vi "Serial Port Clear v0.3.vi"(0 "Serial Port In":i32(ring) items=["Modem Port", "Printer Port", "Serial Card Port #1", "Serial Card Port #2", "Serial Card Port #3", "Serial Card Port #4"]) -> (1 "Serial Port Out":i32(ring) items=["Modem Port", "Printer Port", "Serial Card Port #1", "Serial Card Port #2", "Serial Card Port #3", "Serial Card Port #4"], 2 "string read":string)   [LabVIEW 2020]
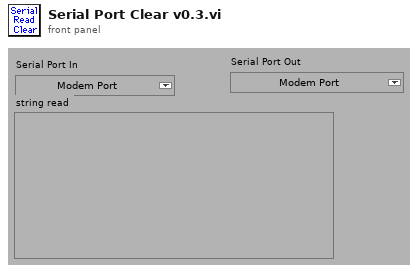
[diagram p1: front panel]
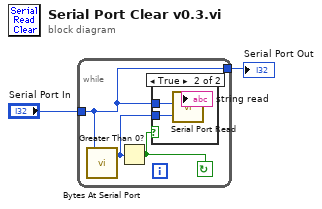
[diagram p0: block diagram]
diagram:
  n1 = while {
    tunnel: [w3] -> w1
    tunnel: "Serial Port In" -> [w3]
    stop <- w5 continue-if-true
    n2 = call <vilib>:"Bytes At Serial Port.vi"("port number"=w3) -> ("byte count"=w4:u32)  [unwired: 1 out]
    n3 = Greater Than 0?(x=w4) -> (x > 0?=w5:bool)
    n4 = case shown="True" w5 {
      tunnel: w4 -> [_ w8]
      tunnel: w3 -> [_ w7]
      frame False {
      }
      frame True {
        n5 = call <vilib>:"Serial Port Read.vi"("requested byte count"=w8, "port number"=w7) -> ("string read"=→"string read":string)  [unwired: 1 out]
      }
    }
  }
  "Serial Port Out" <- w1
